vi "Save Library.vi"(8 "error in (no error)":errorcluster, 10 "Save Path (empty)":path, 11 "Library in":refnum<vi>) -> (0 "error out":errorcluster, 3 "Library out":refnum<vi>)   [LabVIEW 2020, in "gRPC Scripting Tools.lvlib"]
uses:
  gRPC Scripting Tools.lvlib
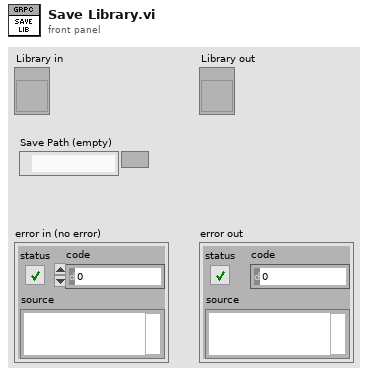
[diagram p1: front panel]
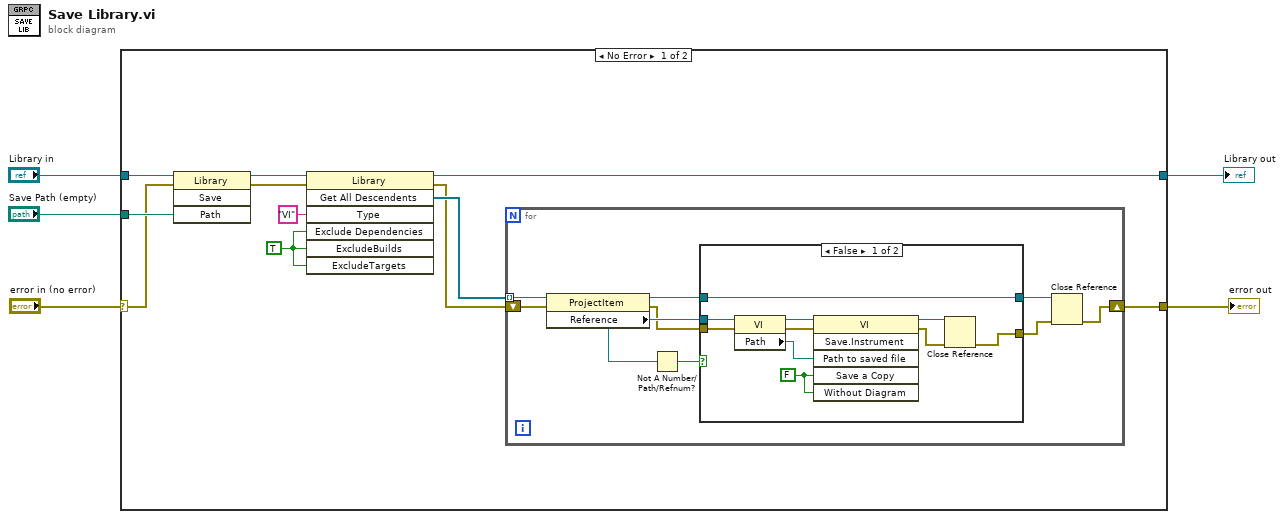
[diagram p0: block diagram]
diagram:
  n1 = case shown="No Error" "error in (no error)" {
    selector: "error in (no error)" -> [w14 w38]
    tunnel: [w6 w38] -> w5
    tunnel: [w12 w39] -> w4
    tunnel: "Library in" -> [w16 w39]
    tunnel: "Save Path (empty)" -> [w15 _]
    frame No Error {
      w9 = TRUE ("ExcludeBuilds")
      n2 = invoke class="Library" method="Save"(reference=w16, error in=w14, "Path"=w15) -> (reference out=w13:refnum<vi>, error out=w11:errorcluster)  [unwired: 1 in, 2 out]
      n3 = invoke class="Library" method="Get All Descendents"(reference=w13, error in=w11, "Type"="VI", "Exclude Dependencies"=w9, "ExcludeBuilds"=w9, "ExcludeTargets"=w9) -> (reference out=w12:refnum<vi>, error out=w7:errorcluster, "All Descendents"=w8:refnum<vi>[])  [unwired: 1 in, 4 out]
      n4 = for {
        tunnel: w8 -> [w25] mode=indexing
        shift-right: [w17] -> w6
        shift-left: w7 -> [w24]
        n5 = property class="ProjectItem"(reference=w25, error in=w24) -> (reference out=w23:refnum<vi>, error out=w20:errorcluster, "Reference"=w21:refnum<vi>)
        n6 = Not A Number/Path/Refnum?(number/path/refnum=w21) -> (NaN/Path/Refnum?=w22:bool)
        n7 = case shown="False" w22 {
          tunnel: [w29 w36] -> w18
          tunnel: w23 -> [w28 w37]
          tunnel: w21 -> [w30 _]
          tunnel: [w28 w37] -> w19
          tunnel: w20 -> [w27 w36]
          frame False {
            w33 = FALSE ("Save a Copy")
            n8 = property class="VI"(reference=w30, error in=w27) -> (reference out=w35:refnum<vi>, error out=w34:errorcluster, "Path"=w26:path)
            n9 = invoke class="VI" method="Save.Instrument"(reference=w35, error in=w34, "Path to saved file"=w26, "Save a Copy"=w33, "Without Diagram"=w33) -> (reference out=w32:refnum<vi>, error out=w31:errorcluster)  [unwired: 1 in, 4 out]
            n10 = Close Reference(reference=w32, error in (no error)=w31) -> (error out=w29:errorcluster)
          }
          frame True {
          }
        }
        n11 = Close Reference(reference=w19, error in (no error)=w18) -> (error out=w17:errorcluster)
      }
    }
    frame Error {
    }
  }
  "error out" <- w5
  "Library out" <- w4
